vi "asset.get.vi"(8 "error in":errorcluster, 11 "Client in":refnum<class "Client.lvclass">) -> (0 "error out":errorcluster, 3 "Client out":refnum<class "Client.lvclass">)   [LabVIEW 2020, in "Client.lvclass"]
doc: "Fetches the asset with the given RID and returns a handle to it."
uses:
  Client.lvclass
  client.lvlib
panel:
  out "out_asset out":i32
  in  "rid":string
  in  "out_asset":i32
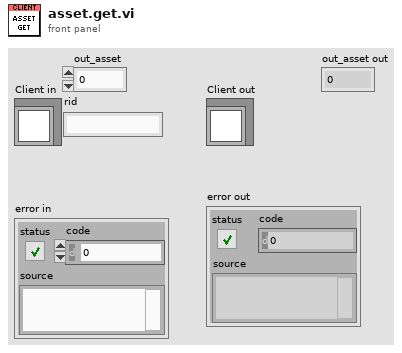
[diagram p1: front panel]
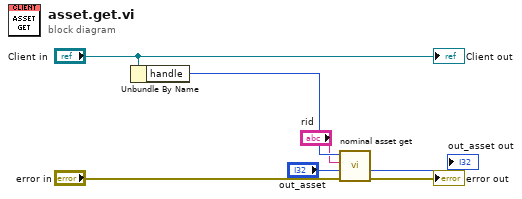
[diagram p0: block diagram]
diagram:
  n1 = Unbundle By Name("Client in") -> ("handle"=w5:i32)
  n2 = call "nominal asset get.vi"("error in (no error)"="error in", "out_asset"="out_asset", "rid"="rid", "client"=w5) -> ("error out"=→"error out":errorcluster, "out_asset out"=→"out_asset out":i32)  [unwired: 5 in, 1 out]
  "Client out" <- "Client in"
